vi "LPF.vi"() -> ()   [LabVIEW 2024]
panel:
  in  "Frequency":dbl=10.0
  in  "Noise amplitude":dbl=0.6
  in  "Lower Cut-Off":dbl=1500.0
  in  "stop":bool
  out "Waveform Chart 2":dynamicdata(graph)
  out "Waveform Chart":dynamicdata(graph)
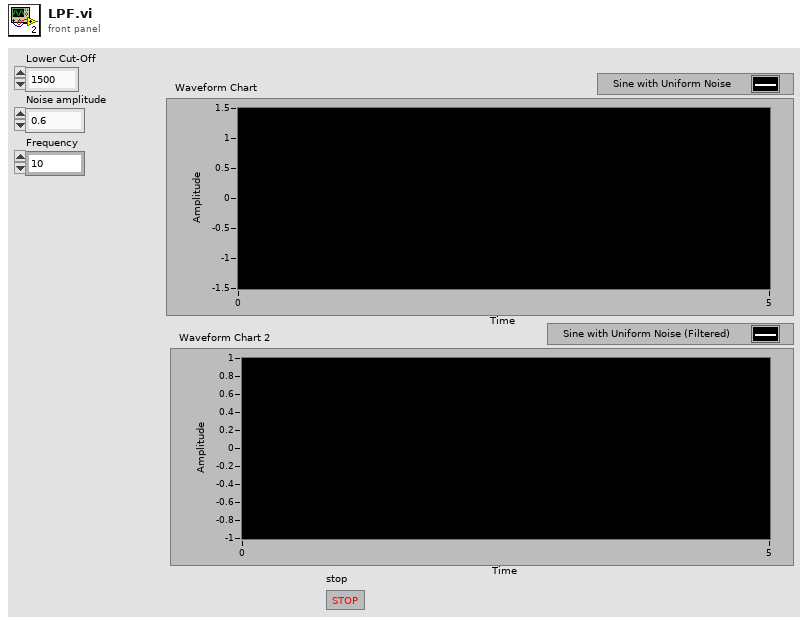
[diagram p1: front panel]
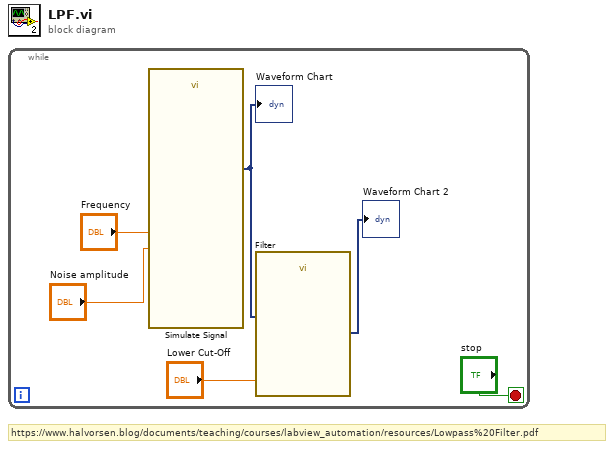
[diagram p0: block diagram]
diagram:
  # "https://www.halvorsen.blog/documents/teaching/courses/labview_automation/resources/Lowpass%20Filter.pdf"
  n1 = while {
    stop <- "stop" stop-if-true
    n2 = call "Simulate Signal"("Frequency"="Frequency", "Noise amplitude"="Noise amplitude") -> ("Sine with Uniform Noise"=w6:dynamicdata)  [unwired: 12 in, 1 out]
    "Waveform Chart" <- w6
    n3 = call "Filter"("Lower Cut-Off"="Lower Cut-Off", "Signal"=w6) -> ("Filtered Signal"=→"Waveform Chart 2":dynamicdata)  [unwired: 8 in, 1 out]
  }
